vi "Update Tree.vi"(8 "error in (no error)":errorcluster, 10 "Tree":refnum<vi>, 11 "OpenHW in":refnum<class "OpenHW.lvclass">) -> (0 "error out":errorcluster, 3 "OpenHW out":refnum<class "OpenHW.lvclass">)   [LabVIEW 2022 SP3, in "open-hw-mon-lv.lvlib" / "OpenHW.lvclass"]
uses:
  OpenHW.lvclass
  OpenHW.lvclass/OpenHW.ctl
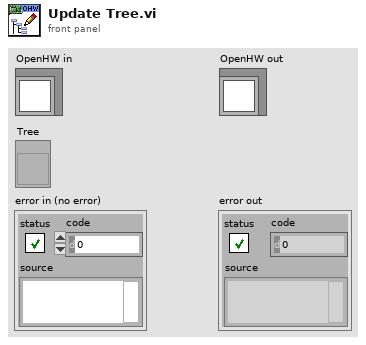
[diagram p1: front panel]
types:
  T1 = typedef "open-hw-mon-lv.lvlib/OpenHW.lvclass/HW Node.ctl" = cluster{"Index":i32, "Text":string, "Value":string, "Min":string, "Max":string, "Parent":i32, "Children":i32[], "ImageURL":string, "Depth":i32}
  T2 = cluster{"Left Cell String":string, "Child Text":string[], "Child Tag":string, "Item Indent":i32, "Child Only?":bool, "Glyph Index":i32}
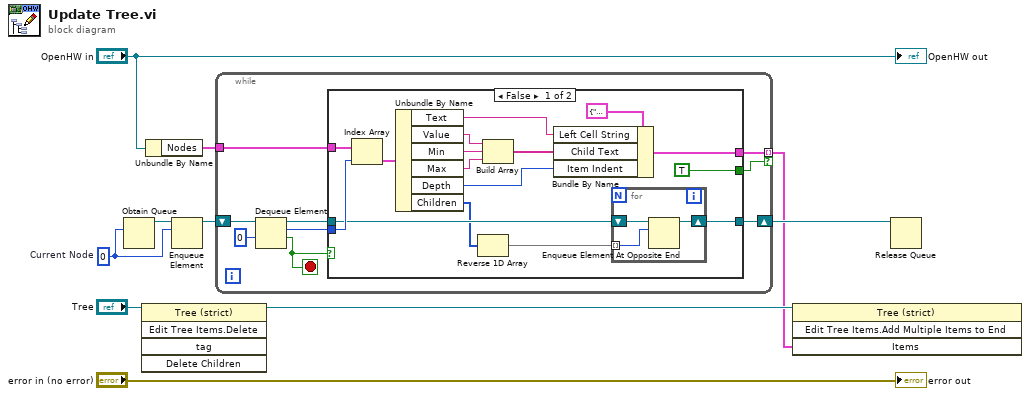
[diagram p0: block diagram]
diagram:
  w6 = 0  # Current Node
  n1 = Obtain Queue(element data type=w6) -> (queue out=w7:refnum<queue>)  [unwired: 4 in, 2 out]
  n2 = invoke on="Invoke Node" class="Tree (strict)" method="Edit Tree Items.Delete"(reference="Tree") -> (reference out=w2:refnum<vi>)  [unwired: 4 in, 4 out]
  n3 = Unbundle By Name("OpenHW in") -> ("Nodes"=w5:T1[])
  n4 = Enqueue Element(queue=w7, element=w6) -> (queue out=w4:refnum<queue>)  [unwired: 2 in, 2 out]
  n5 = while {
    tunnel: w5 -> [w17]
    shift-right: [w14] -> w3
    shift-left: w4 -> [w19]
    tunnel: [w12] -> w1 mode=indexing if=w11
    stop <- w15 stop-if-true
    n6 = Dequeue Element(queue=w19, timeout in ms (-1)=0) -> (queue out=w16:refnum<queue>, element=w13:i32, timed out?=w15:bool)  [unwired: 1 in, 1 out]
    n7 = case shown="False" w15 {
      tunnel: w17 -> [w35 _]
      tunnel: w16 -> [w29 w39]
      tunnel: [w28 w39] -> w14
      tunnel: w13 -> [w34 _]
      tunnel: [w21 _] -> w12
      tunnel: [TRUE _] -> w11
      frame False {
        n8 = Index Array(array=w35, index=w34) -> (element=w33:T1)
        n9 = Unbundle By Name(w33) -> ("Text"=w24:string, "Value"=w31:string, "Min"=w32:string, "Max"=w30:string, "Depth"=w22:i32, "Children"=w27:i32[])
        n10 = Reverse 1D Array(array=w27) -> (reversed array=w26:i32[])
        n11 = Build Array(w31, w32, w30) -> (w23:string[])
        n12 = Bundle By Name(cluster=T2 {"Left Cell String"="", "Child Text"=[], "Child Tag"="", "Item Indent"=0, "Child Only?"=FALSE, "Glyph Index"=0} ("Item"), "Left Cell String"=w24, "Child Text"=w23, "Item Indent"=w22) -> (w21:T2)
        n13 = for {
          shift-right: [w37] -> w28
          shift-left: w29 -> [w38]
          tunnel: w26 -> [w36] mode=indexing
          n14 = Enqueue Element At Opposite End(queue=w38, element=w36) -> (queue out=w37:refnum<queue>)  [unwired: 2 in, 2 out]
        }
      }
      frame True {
      }
    }
  }
  n15 = invoke on="Invoke Node" class="Tree (strict)" method="Edit Tree Items.Add Multiple Items to End"(reference=w2, "Items"=w1) -> ()  [unwired: 2 in, 4 out]
  n16 = Release Queue(queue=w3) -> ()  [unwired: 2 in, 3 out]
  "error out" <- "error in (no error)"
  "OpenHW out" <- "OpenHW in"
